vi "create new file.vi"(10 "File Path":path=path "D:/Data", 11 "Barcode":string) -> ()   [LabVIEW 2015]
uses:
  <vilib>/Utility/file.llb/Write To Spreadsheet File (string).vi
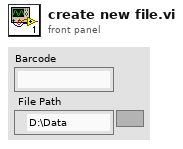
[diagram p1: front panel]
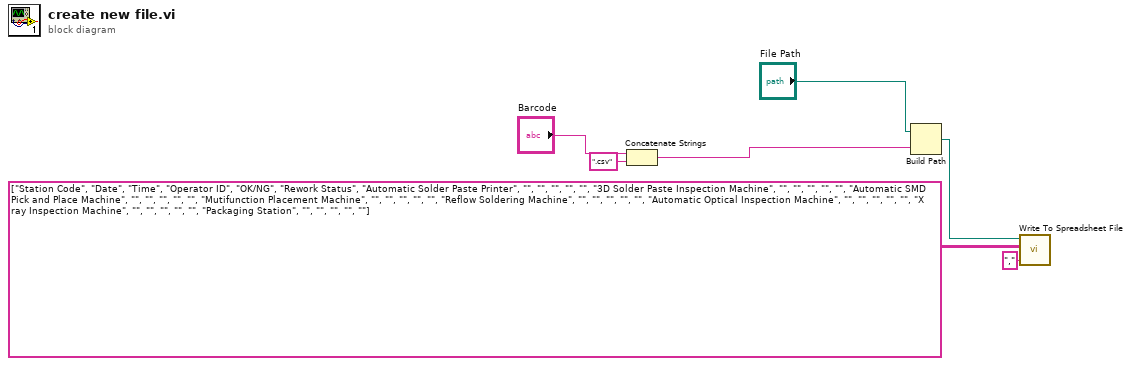
[diagram p0: block diagram]
diagram:
  n1 = Concatenate Strings("Barcode", ".csv" ("string")) -> (w3:string)
  n2 = Build Path(base path="File Path", name or relative path=w3) -> (appended path=w5:path)
  n3 = call-poly <vilib>:"Write To Spreadsheet File.vi"("delimiter (\\t)"="," ("delimiter (\\t)"), "2D data"=string[][] [["Station Code", "Date", "Time", "Operator ID", "OK/NG", "Rework Status"], ["Automatic Solder Paste Printer", "", "", "", "", ""], ["3D Solder Paste Inspection Machine", "", "", "", "", ""], ["Automatic SMD Pick and Place Machine", "", "", "", "", ""], ["Mutifunction Placement Machine", "", "", "", "", ""], ["Reflow Soldering Machine", "", "", "", "", ""], ["Automatic Optical Inspection Machine", "", "", "", "", ""], ["X ray Inspection Machine", "", "", "", "", ""], ["Packaging Station", "", "", "", "", ""]], "file path (dialog if empty)"=w5) -> ()  [unwired: 5 in, 1 out]
